vi "push button and LED.vi"() -> ()   [LabVIEW 2017]
panel:
  in  "Boolean 2":bool
  out "Boolean":bool
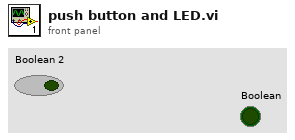
[diagram p1: front panel]
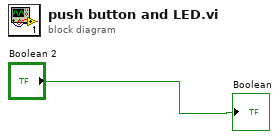
[diagram p0: block diagram]
diagram:
  "Boolean" <- "Boolean 2"
